vi "Fade In.vi"(6 "Fade (Exponential)":T1, 8 "error in":errorcluster, 10 "Fade time (ms)":variant, 11 "VI Reference (calling VI)":refnum<vi>) -> (0 "error out":errorcluster, 3 "dup VI Reference":refnum<vi>)   [LabVIEW 2012]
doc: "Produces a \"Fade In\" on the VI from which a reference has been provided.\n\nVariant (%) can be a numeric or a string containing a number. This allows the use of string-based arguments without the need to convert to a number."
uses:
  _fadetype.ctl
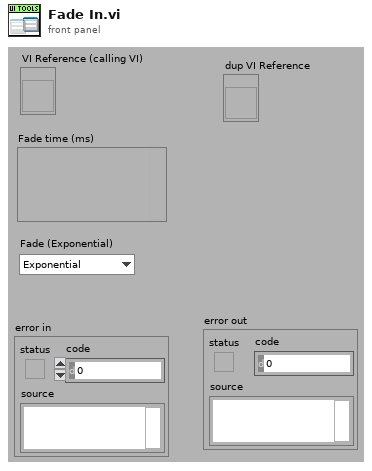
[diagram p1: front panel]
types:
  T1 = typedef "_fadetype.ctl" = enum16{"Exponential", "Linear"}
  T2 = typedef "Type Descriptor Enumeration__ogtk.ctl" = enum8{"<Null>", "I8", "I16", "I32", "I64", "U8", "U16", "U32", "U64", "SGL", "DBL", "EXT", "CSG", "CDB", "CXT", "0x0F", "0x10", "0x11", "0x12", "0x13", "0x14", "Enum U8", "Enum U16", "Enum U32", "Enum U64", "SGL PQ", "DBL PQ", "EXT PQ", "CSG PQ", "CDB PQ", "CXT PQ", "0x1F", "0x20", "Boolean", "0x22", "0x23", "0x24", "0x25", "0x26", "0x27", "0x28", "0x29", "0x2A", "0x2B", "0x2C", "0x2D", "0x2E", "0x2F", "String", "0x31", "Path", "Pict", "0x34", "0x35", "0x36", "DAQ", "0x38", "0x39", "0x3A", "0x3B", "0x3C", "0x3D", "0x3E", "0x3F", "Array", "0x41", "0x42", "0x43", "0x44", "0x45", "0x46", "0x47", "0x48", "0x49", "0x4A", "0x4B", "0x4C", "0x4D", "0x4E", "0x4F", "Cluster", "0x51", "0x52", "Variant", "Waveform", "0x55", "0x56", "0x57", "0x58", "0x59", "0x5A", "0x5B", "0x5C", "0x5D", "0x5E", "0x5F", "0x60", "0x61", "0x62", "0x63", "0x64", "0x65", "0x66", "0x67", "0x68", "0x69", "0x6A", "0x6B", "0x6C", "0x6D", "0x6E", "0x6F", "Refnum"}
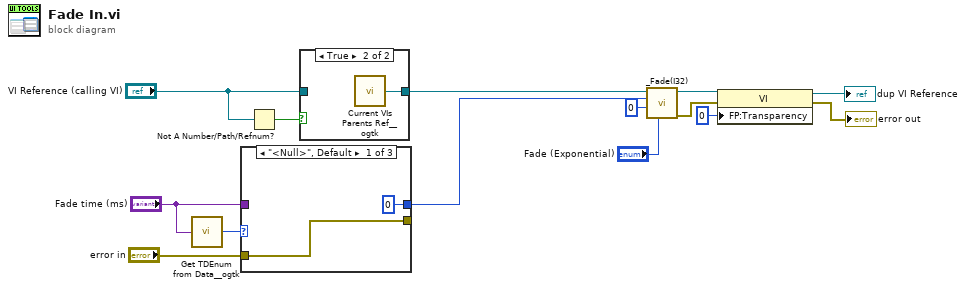
[diagram p0: block diagram]
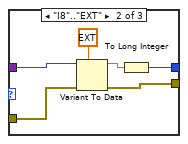
[diagram p3: hidden frame]
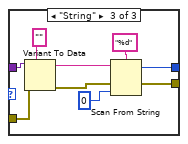
[diagram p4: hidden frame]
diagram:
  n1 = call <userlib>:"Get TDEnum from Data__ogtk.vi"("Data"="Fade time (ms)") -> ("Type Descriptor Enumeration"=w11:T2)  [unwired: 4 out]
  n2 = case shown="\"<Null>\", Default" w11 {
    tunnel: "Fade time (ms)" -> [_ w22 w31]
    tunnel: [0 w19 w28] -> w1
    tunnel: [w15 w18 w23] -> _
    tunnel: "error in" -> [w15 w17 w24]
    frame "<Null>", Default {
    }
    frame "I8".."EXT" {
      n3 = Variant To Data(error in=w17, type=ext 0.0 ("Front Panel Window:Transparency"), Variant=w22) -> (data=w20:ext, error out=w18:errorcluster)
      n4 = To Long Integer(number=w20) -> (32bit integer=w19:i32)
    }
    frame "String" {
      n5 = Variant To Data(error in=w24, type="" ("Front Panel Window:Transparency"), Variant=w31) -> (data=w25:string, error out=w26:errorcluster)
      n6 = Scan From String(format string="%d", input string=w25, error in=w26, default 1=0 ("Front Panel Window:Transparency")) -> (error out=w23:errorcluster, output 1=w28:i32)  [unwired: 1 in, 2 out]
    }
  }
  n7 = Not A Number/Path/Refnum?(number/path/refnum="VI Reference (calling VI)") -> (NaN/Path/Refnum?=w13:bool)
  n8 = case shown="True" w13 {
    tunnel: "VI Reference (calling VI)" -> [w32 _]
    tunnel: [w32 w33] -> w2
    frame False {
    }
    frame True {
      n9 = call <userlib>:"Current VIs Parents Ref__ogtk.vi"() -> ("Calling VI's Reference"=w33:refnum<vi>)  [unwired: 2 out]
    }
  }
  n10 = call "_Fade(I32).vi"("Fade (Exponential)"="Fade (Exponential)", "Target Transparency (0)"=u8 0, "Fade time (ms)"=w1, "VI Reference (calling VI)"=w2) -> ("error out"=w6:errorcluster, "dup VI Reference"=w7:refnum<vi>)  [unwired: 1 in, 5 out]
  n11 = property class="VI"(reference=w7, error in=w6, "FP:Transparency"=u8 0 ("Front Panel Window:Transparency")) -> (reference out=→"dup VI Reference":refnum<vi>, error out=→"error out":errorcluster)
